vi "Read-all-gui-params.vi"(8 "error in (no error)":errorcluster, 11 "Config. params. ref. in":refnum<data-value>) -> (0 "error out":errorcluster, 2 "Configuration params.":T1={"Number of cameras"=1, "Camera 1 port"=enum."B", "ROI width"=0, "ROI height"=1248, "Reset ROI"=FALSE, "Width scale"=0.05, "Height scale"=0.05, "Center Y cam. 1"=0, "Center X cam. 1"=541, "Center Y cam. 2"=624, "Center X cam. 2"=541} {"Center X cam. 2" min=4 max=1244 step=8; "Center Y cam. 2" min=1 max=1082 step=1; "Center X cam. 1" min=4 max=1244 step=8; "Center Y cam. 1" min=1 max=1082 step=1; "Height scale" min=0.001 step=0.001 format="%.3f"; "Width scale" min=0.001 step=0.001 format="%.3f"; "Number of cameras" min=1 max=2 step=1; "ROI width" min=8 max=1248 step=8; "ROI height" min=1 max=1082 step=1}, 3 "Config. params. ref.":refnum<data-value>)   [LabVIEW 2013, in "CameraVision.lvlib" / "CV-Configuration.lvclass"]
uses:
  CV-Configuration.lvclass
  Configuration-parameters-gui.ctl
  CV-Configuration.lvclass/CV-Configuration.ctl
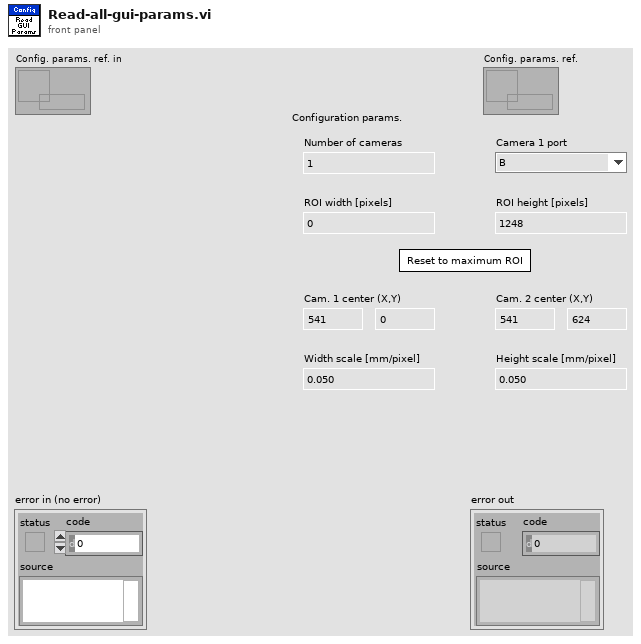
[diagram p1: front panel]
types:
  T1 = typedef "CameraVision.lvlib/CV-Configuration.lvclass/Configuration-parameters-gui.ctl" = cluster{"Number of cameras":i32, "Camera 1 port":enum16{"A", "B"}, "ROI width":u32, "ROI height":u32, "Reset ROI":bool, "Width scale":dbl, "Height scale":dbl, "Center Y cam. 1":i32, "Center X cam. 1":i32, "Center Y cam. 2":i32, "Center X cam. 2":i32}
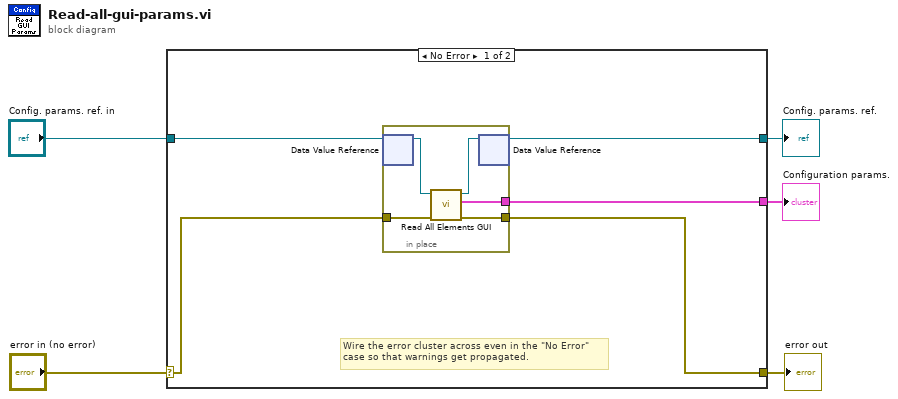
[diagram p0: block diagram]
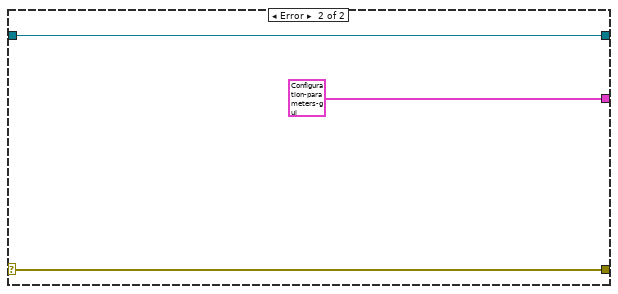
[diagram p2: hidden frame]
diagram:
  n1 = case shown="No Error" "error in (no error)" {
    selector: "error in (no error)" -> [w8 w18]
    tunnel: [w10 w18] -> w4
    tunnel: "Config. params. ref. in" -> [w7 w16]
    tunnel: [w9 T1 {"Number of cameras"=0, "Camera 1 port"=enum."B", "ROI width"=0, "ROI height"=1248, "Reset ROI"=FALSE, "Width scale"=0.0, "Height scale"=0.05, "Center Y cam. 1"=0, "Center X cam. 1"=541, "Center Y cam. 2"=624, "Center X cam. 2"=541} ("Configuration params.")] -> w2
    tunnel: [w6 w16] -> w1
    frame No Error {
      # "Wire the error cluster across even in the \"No Error\"\ncase so that warnings get propagated."
      n2 = in-place {
        in-place-border: [w15] -> w10
        in-place-border: [w14] -> w9
        in-place-border: w8 -> [w13]
        n3 = in-place-dvr #1(w7) -> (w12:refnum<class "CV-Configuration.lvclass">)  [unwired: 1 out]
        n4 = call "Read All Elements GUI.vi"("error in (no error)"=w13, "Config params in"=w12) -> ("error out"=w15:errorcluster, "Configuration params."=w14:T1, "Config params out"=w11:refnum<class "CV-Configuration.lvclass">)  [unwired: 7 in]
        n5 = in-place-dvr #1(w11) -> (w6:refnum<data-value>)  [unwired: 1 out]
      }
    }
    frame Error {
    }
  }
  "error out" <- w4
  "Configuration params." <- w2
  "Config. params. ref." <- w1
